vi "Laser-Read-Energy.vi"(3 "Transimission":i16 min=0 max=100, 4 "error in (no error)":errorcluster, 5 "VISA resource name":refnum<visa-resource-name>) -> (0 "LaserEnergy uJ":dbl, 1 "error out":errorcluster, 2 "VISA resource name out":refnum<visa-resource-name>)   [LabVIEW 2013]
panel:
  out "Energy":string
  out "ReturnState":string
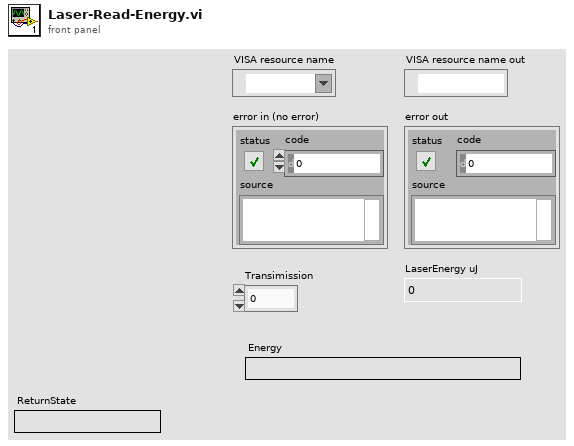
[diagram p1: front panel]
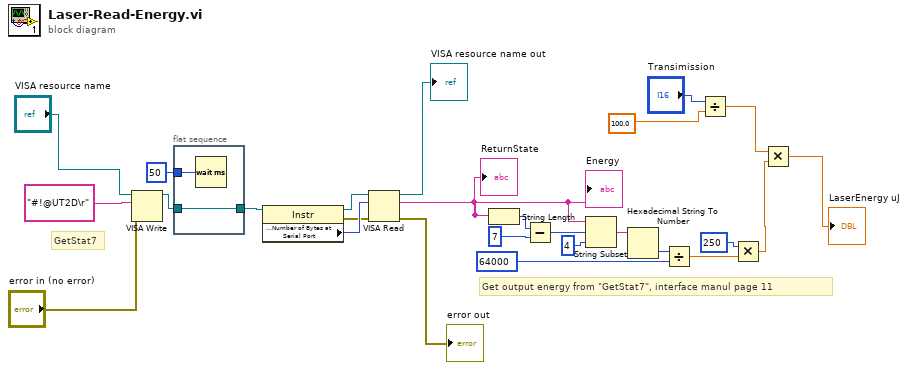
[diagram p0: block diagram]
diagram:
  # "Get output energy from \"GetStat7\", interface manul page 11"
  # "GetStat7"
  n1 = VISA Write(VISA resource name="VISA resource name", write buffer="#!@UT2D\r", error in (no error)="error in (no error)") -> (VISA resource name out=w21:refnum<visa-resource-name>)  [unwired: 2 out]
  n2 = flat-sequence {
    tunnel: w21 -> [w27]
    tunnel: [w27] -> w22
    tunnel: u32 50 ("delay before read (ms)") -> [w28]
    frame #0 {
      n3 = Wait (ms)(milliseconds to wait=w28) -> ()  [unwired: 1 out]
    }
  }
  n4 = property class="Instr"(reference=w22) -> (reference out=w23:refnum<visa-resource-name>, error out=w24:errorcluster, "Serial Settings:Number of Bytes at Serial Port"=w25:u32)  [unwired: 1 in]
  n5 = VISA Read(VISA resource name=w23, byte count=w25, error in (no error)=w24) -> (VISA resource name out=→"VISA resource name out":refnum<visa-resource-name>, read buffer=w16:string, error out=→"error out":errorcluster)  [unwired: 1 out]
  "ReturnState" <- w16
  "Energy" <- w16
  n6 = String Length(string=w16) -> (length=w19:i32)
  n7 = Subtract(x=w19, y=7) -> (x-y=w17:i32)
  n8 = String Subset(string=w16, offset (0)=w17, length (rest)=4) -> (substring=w14:string)
  n9 = Hexadecimal String To Number(string=w14) -> (number=w13:u32)  [unwired: 2 in, 1 out]
  n10 = Divide(x=w13, y=u32 64000) -> (x/y=w11:dbl)
  n11 = Divide(x="Transimission", y=100.0) -> (x/y=w6:dbl)
  n12 = Multiply(x=250, y=w11) -> (x*y=w5:dbl)
  n13 = Multiply(x=w6, y=w5) -> (x*y=→"LaserEnergy uJ":dbl)
